vi "Set View Control Reference.vi"(8 "error in (no error)":errorcluster, 10 "View Control":refnum<vi>, 11 "Debug Log View in":refnum<class "Debug Log View.lvclass">) -> (0 "error out":errorcluster, 3 "Debug Log View out":refnum<class "Debug Log View.lvclass">)   [LabVIEW 2020, in "Debug Log View.lvclass"]
uses:
  Debug Log View.lvclass
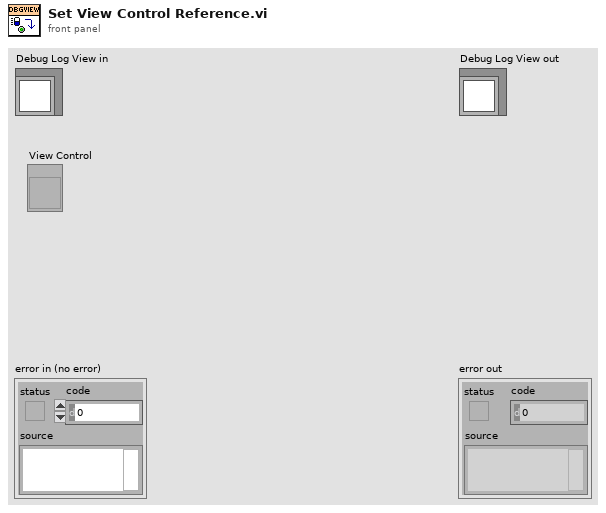
[diagram p1: front panel]
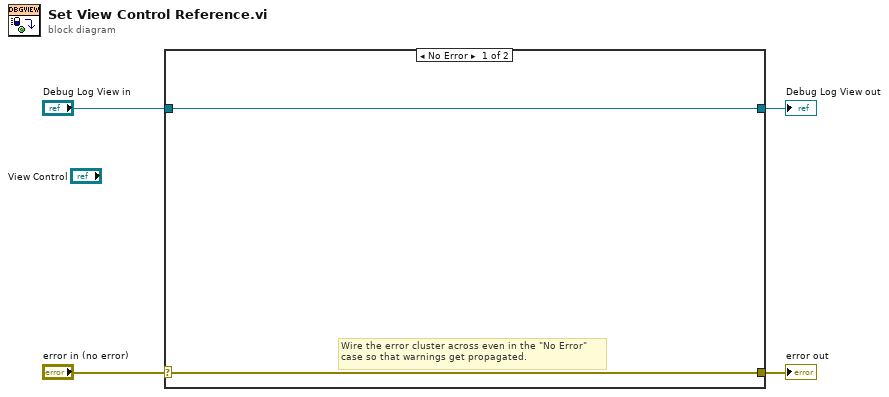
[diagram p0: block diagram]
diagram:
  n1 = case shown="No Error" "error in (no error)" {
    selector: "error in (no error)" -> [w5 w8]
    tunnel: [w5 w8] -> w3
    tunnel: [w6 w7] -> w1
    tunnel: "Debug Log View in" -> [w6 w7]
    frame No Error {
      # "Wire the error cluster across even in the \"No Error\"\ncase so that warnings get propagated."
    }
    frame Error {
    }
  }
  "error out" <- w3
  "Debug Log View out" <- w1
